vi "INIT controllers.vi"(8 "error in (no error)":errorcluster) -> (0 "error out":errorcluster)   [LabVIEW 2023]
uses:
  <vilib>/Rock Robotics/WPI/Joystick/WPI_JoystickDeviceEnum.ctl
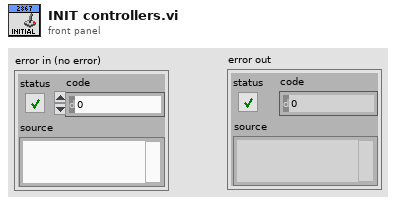
[diagram p1: front panel]
types:
  T1 = typedef "WPI_JoystickDeviceEnum.ctl" = enum16{"USB 0", "USB 1", "USB 2", "USB 3", "USB 4", "USB 5"}
  T2 = typedef "WPI_JoystickDevRef.ctl" = cluster{"Device":T1}
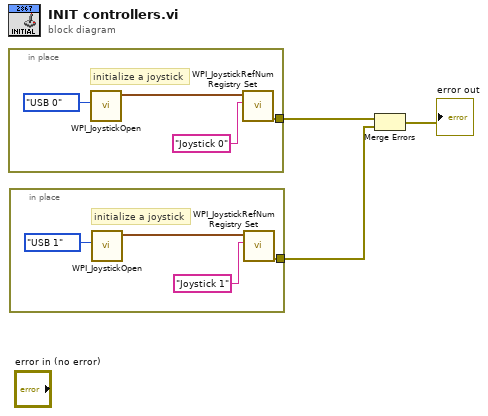
[diagram p0: block diagram]
diagram:
  n1 = in-place {
    in-place-border: [w4] -> w3
    # "initialize a joystick"
    n2 = call <vilib>:"WPI_JoystickOpen.vi"("JoystickDevice"=WPI_JoystickDeviceEnum."USB 0") -> ("JoystickDevRef"=w6:T2)  [unwired: 10 in]
    n3 = call <vilib>:"WPI_JoystickRefNum Registry Set.vi"("refnum name"="Joystick 0", "JoystickDevRef"=w6) -> ("error out"=w4:errorcluster)  [unwired: 8 in, 1 out]
  }
  n4 = in-place {
    in-place-border: [w8] -> w1
    # "initialize a joystick"
    n5 = call <vilib>:"WPI_JoystickOpen.vi"("JoystickDevice"=WPI_JoystickDeviceEnum."USB 1") -> ("JoystickDevRef"=w10:T2)  [unwired: 10 in]
    n6 = call <vilib>:"WPI_JoystickRefNum Registry Set.vi"("refnum name"="Joystick 1", "JoystickDevRef"=w10) -> ("error out"=w8:errorcluster)  [unwired: 8 in, 1 out]
  }
  n7 = Merge Errors(w3, w1) -> (→"error out":errorcluster)
